vi "836Robot Global Data.vi"() -> ()   [LabVIEW 2011]
doc: "This global VI can contain as many global variables as you need. Place a control on the panel, give it a good name. To read or write to it from a VI, drag the icon to the diagram of that VI. You can also drag from the project. Click on the node to change which global you access. You shouldn't have multiple locations writing to a global or it will cause a race-condition."
uses:
  <vilib>/Rock Robotics/WPI/Camera/WPI_CameraImageSize.ctl
panel:
  out "MiniBot Deploy":bool
  out "Accel Z":dbl
  out "Accel Y":dbl
  out "Accel X":dbl
  out "Visited Disabled":dbl
  out "Visited TeleOp":dbl
  out "Visited Auton":dbl
  out "Disabled Elapsed Seconds":dbl
  out "TeleOp Elapsed Seconds":dbl
  out "Auton Elapsed Seconds":dbl
  out "Battery Voltage":dbl
  out "avg Drive Encoders":dbl
  out "Sonar Distance":dbl
  out "Error X":dbl
  out "Arm Reset":bool
  out "Right Wheel Encoder":dbl
  out "Left Wheel Encoder":dbl
  in  "ArmEncoder":dbl
  out "Bearing To Target":dbl
  out "Camera PV":dbl
  out "Camera Setpoint":dbl
  in  "CrossHair":cluster{"X_CrossHair":i32, "Y_CrossHair":i32}
  out "Selected Target":dbl
  in  "SelectedTargetInfo":T1
  in  "SelectedTargetError":cluster{"ErrorY":i32, "ErrorX":i32}
  out "Available Targets":sgl
  in  "FAILSAFE":bool
  out "Elevator Encoder":dbl
  in  "Close Claw":bool
  in  "Open Claw":bool
  in  "Claw State":T2(ring)
  in  "Gyro Angle":dbl
  in  "LED toggle rate (ms)":u32
  in  "image size":T3=enum."320x240"
  in  "Enable Vision":bool=TRUE
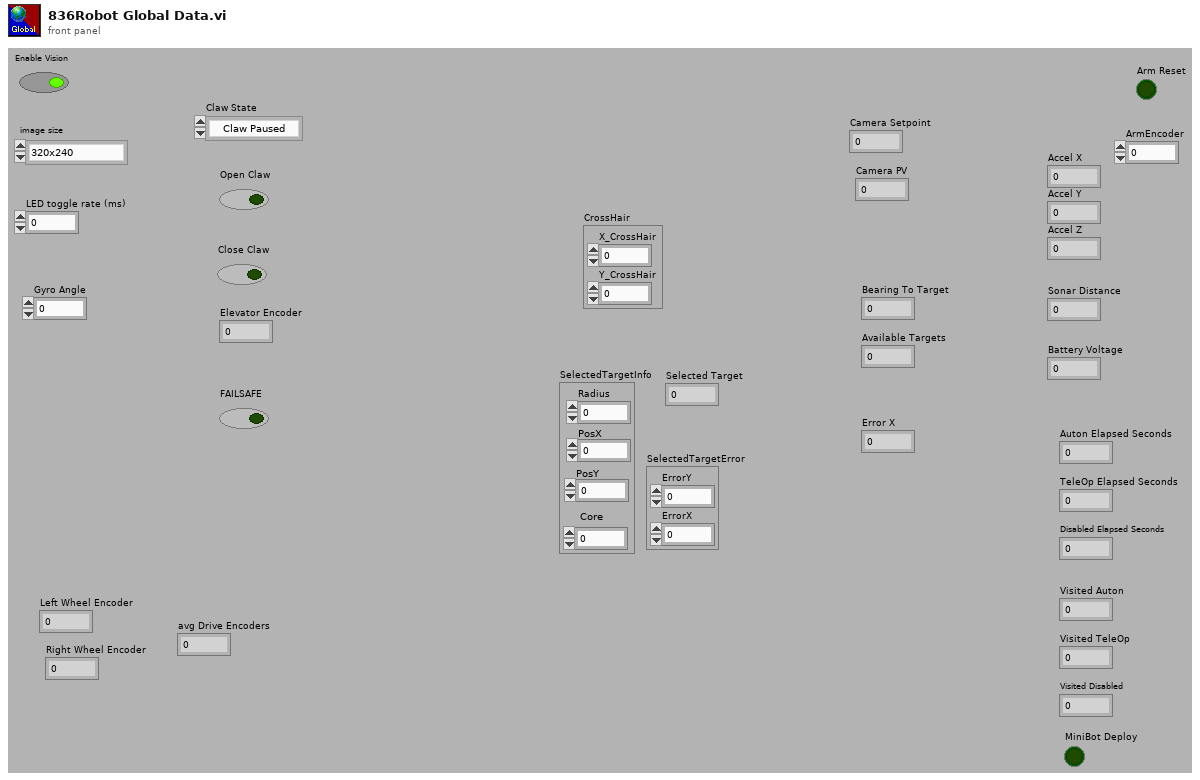
[diagram p1: front panel]
types:
  T1 = cluster{"Radius":i32, "PosX":i32, "PosY":i32, "Core":i32}
  T2 = enum16{"Claw Paused", "Claw Open", "Claw Moving", "Claw Closed"}
  T3 = typedef "WPI_CameraImageSize.ctl" = enum16{"640x480", "320x240", "160x120"}
diagram:
